vi "Send Status Updated.vi"(8 "error in (no error)":errorcluster, 10 "Status":string, 11 "Chat Window UI Controller in":refnum<class "Chat Window UI Controller.lvclass">) -> (0 "error out":errorcluster, 3 "Chat Window UI Controller out":refnum<class "Chat Window UI Controller.lvclass">)   [LabVIEW 2014, in "Chat Window UI Controller.lvlib" / "Chat Window UI Controller.lvclass"]
uses:
  Chat Window UI Controller.lvclass
  Chat Window UI Controller Messages/Status Updated Msg/Status Updated Msg.lvclass
  <vilib>/ActorFramework/Actor/Actor.lvclass
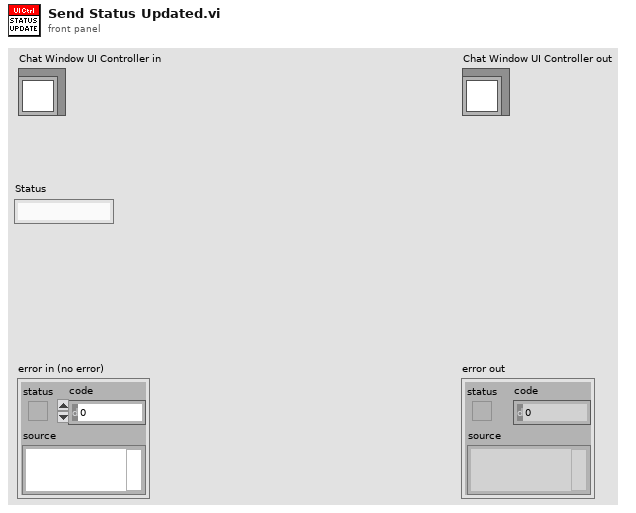
[diagram p1: front panel]
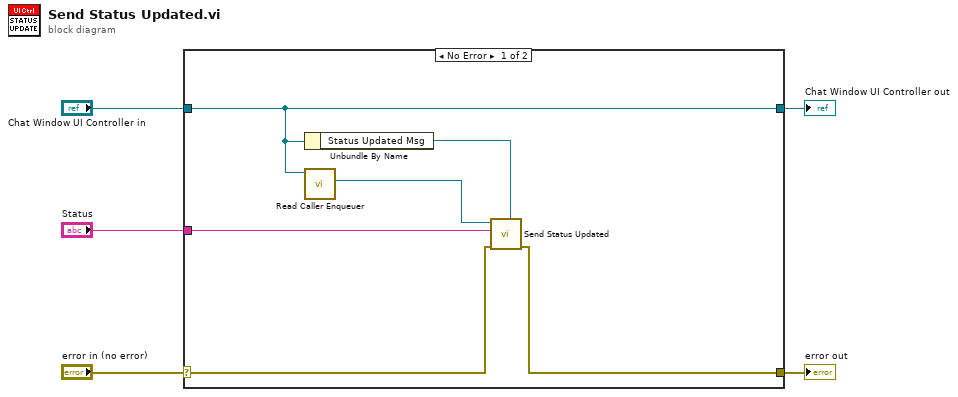
[diagram p0: block diagram]
diagram:
  n1 = case shown="No Error" "error in (no error)" {
    selector: "error in (no error)" -> [w7 w13]
    tunnel: [w6 w13] -> w4
    tunnel: [w10 w12] -> w2
    tunnel: "Chat Window UI Controller in" -> [w10 w12]
    tunnel: "Status" -> [w8 _]
    frame No Error {
      n2 = Unbundle By Name(w10) -> ("Status Updated Msg"=w11:refnum<class "Status Updated Msg.lvclass">)
      n3 = call <vilib>:"Read Caller Enqueuer.vi"("Actor"=w10) -> ("Caller Enqueuer"=w9:refnum<class "Message Enqueuer.lvclass">)  [unwired: 10 in]
      n4 = call "Send Status Updated.vi"("Message Type"=w11, "error in (no error)"=w7, "Status"=w8, "Message Enqueuer"=w9) -> ("error out"=w6:errorcluster)  [unwired: 6 in, 1 out]
    }
    frame Error {
    }
  }
  "error out" <- w4
  "Chat Window UI Controller out" <- w2
